vi "Build intens graph with peaks.vi"(0 "data":dbl[][](array[numeric]), 5 "dates":string[](array[string])) -> (4 "Peaks":cluster{i32[], dbl[]}[](graph), 10 "Peaks":dbl[](array[numeric]), 12 "Max cluster":T2 {"Hour" format="%<%H:%M>t"}, 13 "Min Cluster":T1 {"Hour" format="%<%H:%M>t"}, 14 "%":dbl[](array[numeric]) format="%#_2g", 15 "Intensity Graph":dbl[][](graph))   [LabVIEW 2018]
uses:
  <vilib>/Analysis/NI_AALBase.lvlib
panel:
  out "Waveform Graph 2":dbl[](graph)
  out "index min":i32
  out "index max":i32
  out "min value":dbl
  out "Hour of min":i32 format="%<%H:%M>t"
  out "Hour of peak":i32 format="%<%H:%M>t"
  out "Waveform Graph":dbl[](graph)
  out "Max peak":dbl
  in  "intervals":i32=10
  out "Histogram":cluster{i32[], dbl[]}(graph)
  out "Peaks":dbl[][](graph)
  out "peaks":dbl[][](array[numeric])
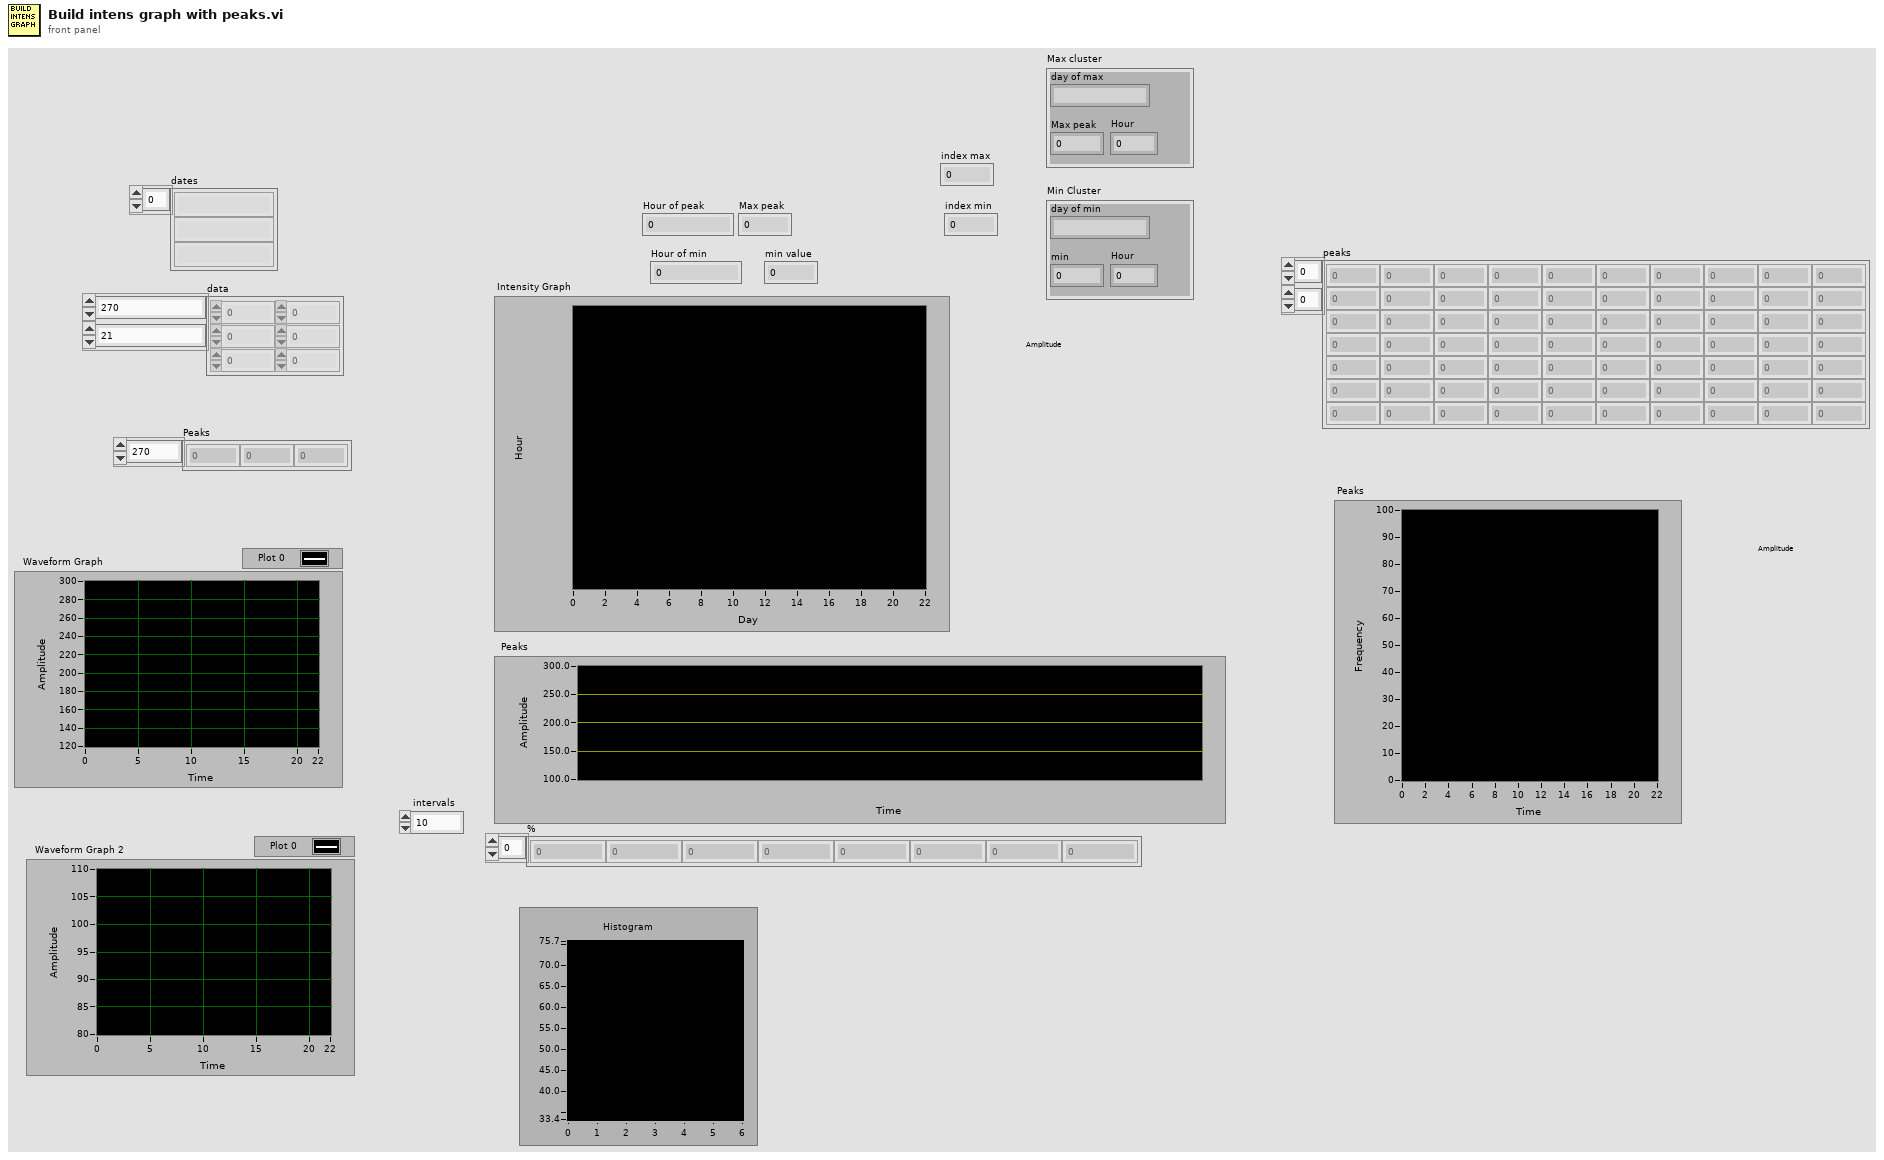
[diagram p1: front panel]
types:
  T1 = cluster{"Hour":i32, "min":dbl, "day of min":string}
  T2 = cluster{"Hour":i32, "Max peak":dbl, "day of max":string}
  T3 = cluster{"Histogram: h(x)":i32[], "X Values":dbl[]}
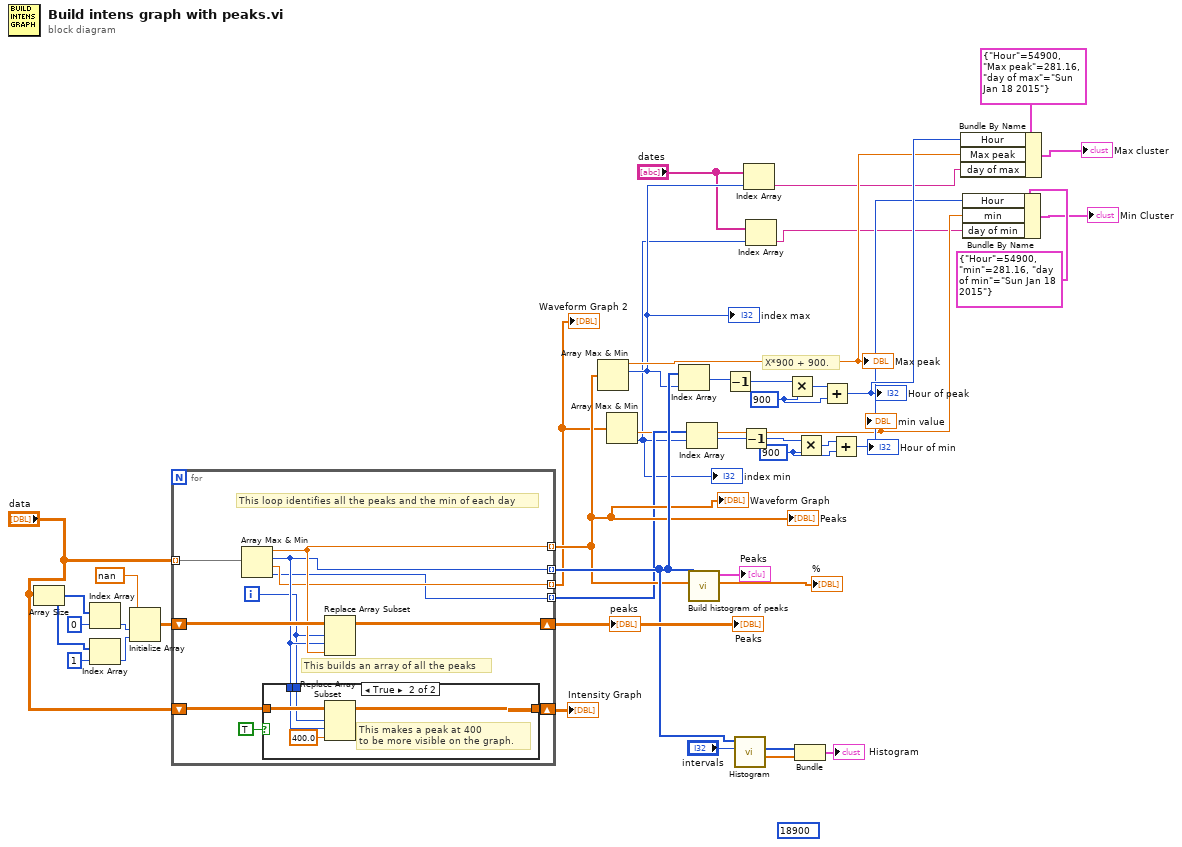
[diagram p0: block diagram]
diagram:
  w20 = 900 ("y")
  (unwired) 18900 ("Hour of peak")
  w21 = 900 ("y")
  # "X*900 + 900."
  n1 = Array Size(array="data") -> (size(s)=w39:i32[])
  n2 = Index Array(array=w39, index=0) -> (element=w37:i32)
  n3 = Index Array(array=w39, index=1) -> (element=w38:i32)
  n4 = Initialize Array(nan, w37, w38) -> (w34:dbl[][])
  n5 = for {
    tunnel: "data" -> [w52] mode=indexing
    shift-right: [w50] -> w35
    shift-left: w34 -> [w51]
    tunnel: [w46] -> w25 mode=indexing
    tunnel: [w47] -> w24 mode=indexing
    shift-right: [w49] -> w32
    shift-left: "data" -> [w48]
    tunnel: [w43] -> w14 mode=indexing
    tunnel: [w42] -> w17 mode=indexing
    i -> [w45]
    # "This builds an array of all the peaks"
    # "This loop identifies all the peaks and the min of each day"
    n6 = Array Max & Min(array=w52) -> (max value=w47:dbl, max index (indices)=w46:i32, min value=w43:dbl, min index (indices)=w42:i32)
    n7 = case shown="True" TRUE {
      tunnel: [w53 w58] -> w49
      tunnel: w48 -> [w53 w57]
      tunnel: w46 -> [_ w56]
      tunnel: w45 -> [_ w54]
      frame False {
      }
      frame True {
        # "This makes a peak at 400\nto be more visible on the graph."
        n8 = Replace Array Subset(array=w57, new element=400.0 ("new element/subarray"), index (row)=w54, index (col)=w56) -> (w58:dbl[][])
      }
    }
    n9 = Replace Array Subset(array=w51, new element=w47, index (row)=w45, index (col)=w46) -> (w50:dbl[][])
  }
  "peaks" <- w35
  "Intensity Graph" <- w32
  "Peaks" <- w35
  "Peaks" <- w24
  "Waveform Graph" <- w24
  "Waveform Graph 2" <- w14
  n10 = Array Max & Min(array=w24) -> (max value=w11:dbl, max index (indices)=w10:i32)  [unwired: 2 out]
  "Max peak" <- w11
  "index max" <- w10
  n11 = Array Max & Min(array=w14) -> (min value=w5:dbl, min index (indices)=w3:i32)  [unwired: 2 out]
  "min value" <- w5
  "index min" <- w3
  n12 = Index Array(array=w25, index=w10) -> (element=w23:i32)
  n13 = Index Array(array=w17, index=w3) -> (element=w18:i32)
  n14 = call "Build histogram of peaks.vi"("Peaks"=w24, "Hours of peaks"=w25) -> ("%"=→"%":dbl[], "Peaks"=→"Peaks":cluster{i32[], dbl[]}[])  [unwired: 7 in, 1 out]
  n15 = Decrement(x=w23) -> (x-1=w16:i32)
  n16 = call <vilib>:"Histogram.vi"("intervals"="intervals", "X"=w25) -> ("X Values"=w28:dbl[], "Histogram: h(x)"=w29:i32[])  [unwired: 6 in, 2 out]
  n17 = Decrement(x=w18) -> (x-1=w15:i32)
  n18 = Index Array(array="dates", index=w10) -> (element=w9:string)
  n19 = Index Array(array="dates", index=w3) -> (element=w2:string)
  n20 = Multiply(x=w16, y=w21) -> (x*y=w22:i32)
  n21 = Bundle("Histogram: h(x)"=w29, "X Values"=w28) -> (→"Histogram":T3)  [unwired: 1 in]
  n22 = Multiply(x=w15, y=w20) -> (x*y=w19:i32)
  n23 = Add(x=w22, y=w21) -> (x+y=w12:i32)
  "Hour of peak" <- w12
  n24 = Add(x=w19, y=w20) -> (x+y=w6:i32)
  "Hour of min" <- w6
  n25 = Bundle By Name(cluster=T2 {"Hour"=54900, "Max peak"=281.16, "day of max"="Sun Jan 18 2015"} ("Max cluster"), "Hour"=w12, "Max peak"=w11, "day of max"=w9) -> (→"Max cluster":T2)
  n26 = Bundle By Name(cluster=T1 {"Hour"=54900, "min"=281.16, "day of min"="Sun Jan 18 2015"} ("Min Cluster"), "Hour"=w6, "min"=w5, "day of min"=w2) -> (→"Min Cluster":T1)
